vi "1820 LPF ON duration.vi"(10 "Lambda":bool, 11 "LPF ON":timestamp) -> (3 "LPF on (HH:MM:SS)":dbl format="%<%H:%M:%S>t")   [LabVIEW 2016, in "Instrument.OxfordVRM.lvclass"]
uses:
  Instrument.OxfordVRM.lvclass
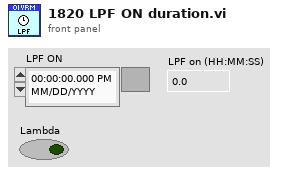
[diagram p1: front panel]
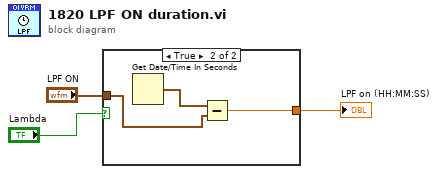
[diagram p0: block diagram]
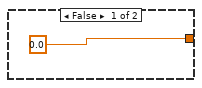
[diagram p2: hidden frame]
diagram:
  n1 = case shown="True" "Lambda" {
    tunnel: "LPF ON" -> [_ w5]
    tunnel: [0.0 ("LPF on (s)") w6] -> w3
    frame False {
    }
    frame True {
      n2 = Get Date/Time In Seconds() -> (seconds since 1Jan1904=w7:timestamp)
      n3 = Subtract(x=w7, y=w5) -> (x-y=w6:dbl)
    }
  }
  "LPF on (HH:MM:SS)" <- w3
